vi "Loop_HW.vi"   [LabVIEW 2017, in "Joystick.lvlib"]
uses:
  Joystick.lvlib
  Globals/Global_STOP.vi
  Globals/Global_Joystick.vi
types:
  T1 = typedef "WPI_JoystickDevRef.ctl" = cluster{"Device":T2}
  T2 = typedef "WPI_JoystickDeviceEnum.ctl" = enum16{"USB 0", "USB 1", "USB 2", "USB 3", "USB 4", "USB 5"}
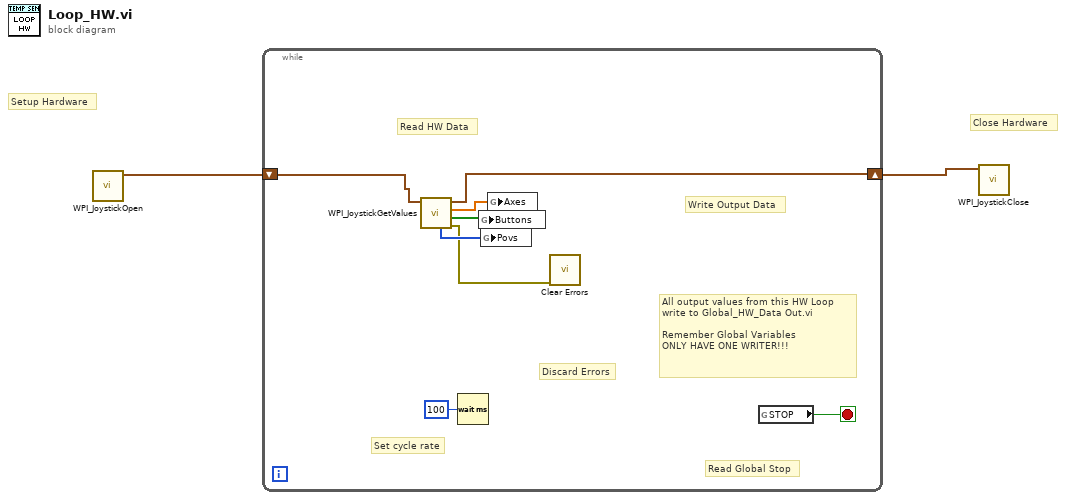
[diagram p0: block diagram]
diagram:
  # "Close Hardware"
  # "Setup Hardware"
  n1 = call <vilib>:"WPI_JoystickOpen.vi"() -> ("JoystickDevRef"=w2:T1)  [unwired: 11 in]
  n2 = while {
    shift-right: [w7] -> w1
    shift-left: w2 -> [w8]
    stop <- w10 stop-if-true
    # "Discard Errors"
    # "All output values from this HW Loop\nwrite to Global_HW_Data Out.vi\n\nRemember Global Variables\nONLY HAVE ONE WRITER!!!"
    # "Read HW Data"
    # "Read Global Stop"
    # "Set cycle rate"
    # "Write Output Data"
    n3 = call <vilib>:"WPI_JoystickGetValues.vi"("JoystickDevRef"=w8) -> ("error out"=w3:errorcluster, "Buttons"=w6:bool[], "Axes"=w5:dbl[], "JoystickDevRef"=w7:T1, "POVs"=w4:i16[])  [unwired: 6 in]
    n4 = Wait (ms)(milliseconds to wait=u32 100) -> ()  [unwired: 1 out]
    n5 = global write "Global_Joystick.vi" "Buttons"(w6) -> ()
    n6 = global write "Global_Joystick.vi" "Povs"(w4) -> ()
    n7 = global write "Global_Joystick.vi" "Axes"(w5) -> ()
    n8 = call <vilib>:"Clear Errors.vi"("error in (no error)"=w3) -> ()  [unwired: 5 in, 2 out]
    n9 = global read "Global_STOP.vi" "STOP"() -> (w10:bool)
  }
  n10 = call <vilib>:"WPI_JoystickClose.vi"("JoystickDevRef"=w1) -> ()  [unwired: 11 in]
